vi "Run.vi"(8 "error in (no error)":errorcluster, 11 "Project in":refnum<class "LabVIEW Build.lvclass">) -> (0 "error out":errorcluster, 2 "Text":string, 3 "Project out":refnum<class "LabVIEW Build.lvclass">)   [LabVIEW 2014, in "LabVIEW Build.lvclass"]
uses:
  LabVIEW Build.lvclass
  LabVIEW Build.lvclass/LabVIEW Build.ctl
  Build Job/Build Job.lvclass/Build Job.ctl
  Build Job/Read Hostname.vi
  Build Job/Read Job Build Info.vi
  Build Job/Read Parameters.vi
  Build Job/Write Parameters.vi
  Build Job/Build Job.lvclass
  <vilib>/wsapi/NI_WebServices.lvlib
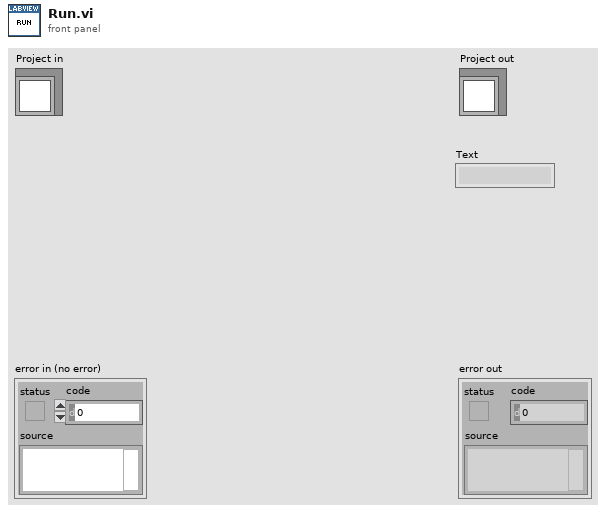
[diagram p1: front panel]
types:
  T1 = typedef "LabVIEW Build - STYP.ctl" = cluster{"Executor_Number":string, "Workspace_Path":string, "Build_Spec":string, "Project_Path":string, "Auto_Version_Increment":bool}
  T2 = typedef "Job Build Info - STYP.ctl" = cluster{"Build Name":string, "Description":string, "Notification":string, "Artifact Days":string, "Project Folder":string}
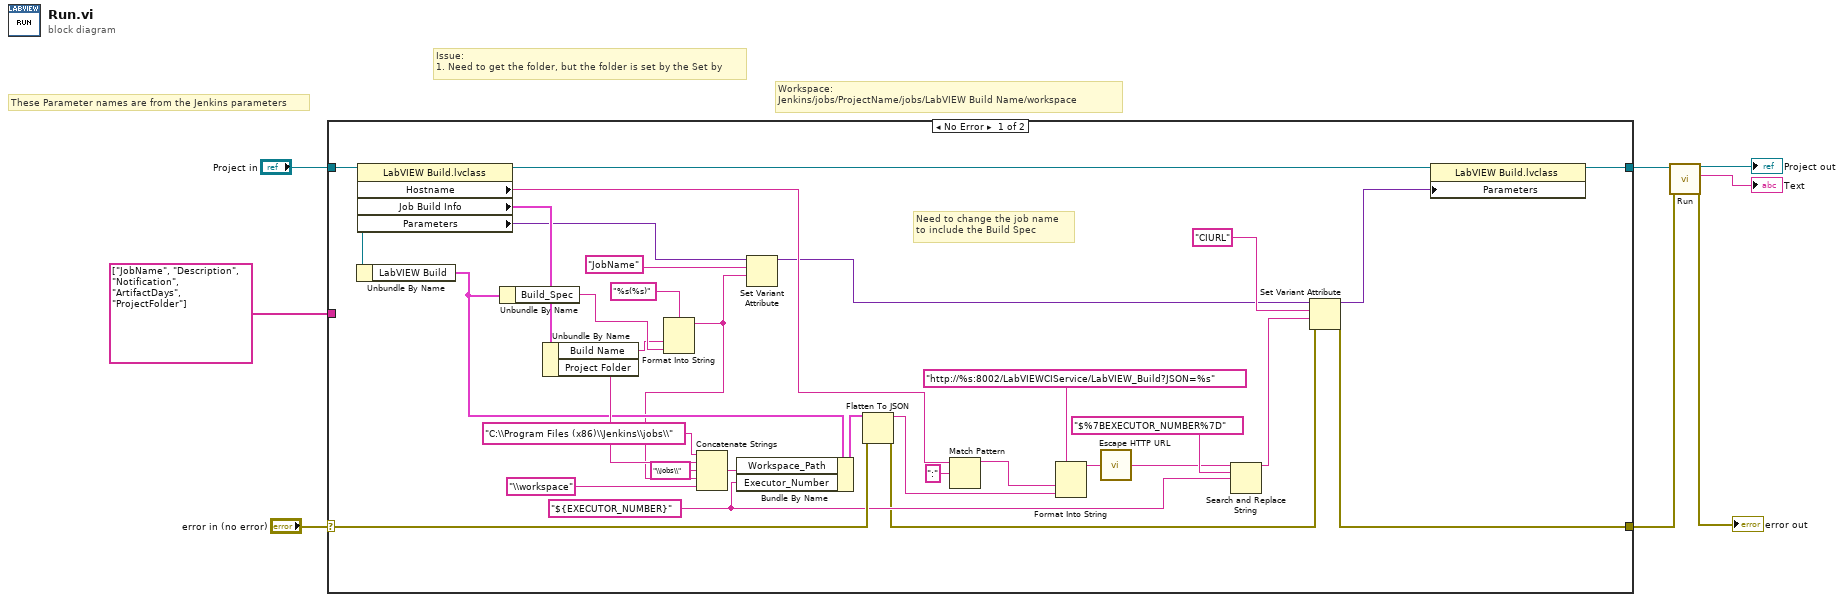
[diagram p0: block diagram]
diagram:
  # "Issue:\n1. Need to get the folder, but the folder is set by the Set by"
  # "Workspace:\nJenkins/jobs/ProjectName/jobs/LabVIEW Build Name/workspace"
  # "These Parameter names are from the Jenkins parameters"
  n1 = case shown="No Error" "error in (no error)" {
    selector: "error in (no error)" -> [w40 w43]
    tunnel: [w17 w43] -> w4
    tunnel: [w41 w42] -> w7
    tunnel: "Project in" -> [w23 w42]
    tunnel: string[] ["JobName", "Description", "Notification", "ArtifactDays", "ProjectFolder"] -> [_ _]
    frame No Error {
      w28 = "${EXECUTOR_NUMBER}" ("Executor_Number")
      # "Need to change the job name\nto include the Build Spec"
      n2 = Unbundle By Name(w23) -> ("LabVIEW Build"=w15:T1)
      n3 = property class="LabVIEW Build.lvclass"(reference=w23) -> (reference out=w22:refnum<class "LabVIEW Build.lvclass">, "Hostname"=w21:string, "Job Build Info"=w20:T2, "Parameters"=w10:variant)  [unwired: 1 in, 1 out]
      n4 = Unbundle By Name(w15) -> ("Build_Spec"=w13:string)
      n5 = Unbundle By Name(w20) -> ("Build Name"=w12:string, "Project Folder"=w19:string)
      n6 = Format Into String(format string="%s(%s)", w12, w13) -> (resulting string=w11:string)  [unwired: 2 in, 1 out]
      n7 = Concatenate Strings("C:\\Program Files (x86)\\Jenkins\\jobs\\" ("format string"), w19, "\\jobs\\" ("string"), w11, "\\workspace" ("string")) -> (w31:string)
      n8 = Bundle By Name(cluster=w15, "Workspace_Path"=w31, "Executor_Number"=w28) -> (w35:T1)
      n9 = Set Variant Attribute(Variant=w10, name="JobName" ("Name"), value=w11) -> (Variant out=w9:variant)  [unwired: 1 in, 2 out]
      n10 = Flatten To JSON(anything=w35, error in (no error)=w40) -> (JSON string=w36:string, 11:w18:errorcluster)  [unwired: 1 in]
      n11 = Match Pattern(string=w21, regular expression=":") -> (before substring=w37:string)  [unwired: 1 in, 3 out]
      n12 = Format Into String(format string="http://%s:8002/LabVIEWCIService/LabVIEW_Build?JSON=%s", w37, w36) -> (resulting string=w34:string)  [unwired: 2 in, 1 out]
      n13 = call <vilib>:"Escape HTTP URL.vi"("unescaped string in"=w34) -> ("escaped string out"=w29:string)
      n14 = Search and Replace String(input string=w29, search string="$%7BEXECUTOR_NUMBER%7D" ("replace string (\"\")"), replace string=w28) -> (result string=w25:string)  [unwired: 5 in, 3 out]
      n15 = Set Variant Attribute(Variant=w9, name="CIURL" ("Name"), value=w25, error in=w18) -> (Variant out=w24:variant, error out=w17:errorcluster)  [unwired: 1 out]
      n16 = property class="LabVIEW Build.lvclass"(reference=w22, "Parameters"=w24) -> (reference out=w41:refnum<class "LabVIEW Build.lvclass">)  [unwired: 1 in, 1 out]
    }
    frame Error {
    }
  }
  n17 = call-parent "Run.vi"("error in (no error)"=w4, "Project in"=w7) -> ("error out"=→"error out":errorcluster, "Text"=→"Text":string, "Project out"=→"Project out":refnum<class "LabVIEW Build.lvclass">)  [unwired: 7 in]
